vi "M2p_AD_Fifo_ToBinaryFile.vi"() -> ()   [LabVIEW 2015]
uses:
  spcm_library/spcm_gui_common.llb/element_device.ctl
  spcm_library/spcm_gui_common.llb/element_mode_fifo.ctl
  spcm_library/spcm_gui_common.llb/element_device_infos.ctl
  spcm_library/spcm_gui_m2p.llb/element_m2p_ai_channel.ctl
  spcm_library/spcm_gui_m2p.llb/element_m2p_clock.ctl
  spcm_library/spcm_gui_m2p.llb/element_m2p_ai_trigger.ctl
panel:
  out "Transferred Samples":u64=666894336
  out "Transferred Samples (MBytes)":u64=636
  in  "File Name":string="stream.dat"
  in  "Trigger Settings":T1={"Trigger Source"=0, "External Trigger"=0, "Level 0 Ext"=1500, "Ext Trig Term"=FALSE, "Channel Trigger"=0, "Level 0 Ch"=0, "Level 1 Ch"=0, "Trigger Delay (Samples)"=0} {"Channel Trigger" items=["None", "Pos. Edge", "Neg. Edge", "Any Edge", "Pos. Rearm", "Neg. Rearm", "Enter Window", "Leave Window", "In Win", "Out Win"]; "External Trigger" items=["None", "Pos. Edge", "Neg. Edge", "Any Edge", "High Level", "Low Level"]; "Trigger Source" items=["Software Trigger", "External Trigger", "Channel 0 Trigger", "Channel 1 Trigger", "Channel 2 Trigger", "Channel 3 Trigger", "Channel 4 Trigger", "Channel 5 Trigger", "Channel 6 Trigger", "Channel 7 Trigger"]; "Trigger Delay (Samples)" max=65535 step=1}
  in  "Clock Settings":T2={"Clock Mode"=0, "Sampling Rate (kHz)"=10000.0, "Clock Output"=FALSE, "Termination"=FALSE, "Ref. Clock (MHz)"=10.0, "Threshold (mV)"=1500} {"Threshold (mV)" min=-5000 max=5000; "Clock Mode" items=["Internal Clock Quartz", "External Clock", "External Reference Clock"]; "Ref. Clock (MHz)" min=0.0 max=125000.0; "Sampling Rate (kHz)" min=1.0 max=5000000.0}
  in  "AI Channel 7":T3={"Enable"=TRUE, "Input Range "=2, "Termination"=0, "Input Type"=0, "Offset"=0} {"Input Type" items=["Single-ended", "Differential"]; "Termination" items=["1 MOhm", "50 Ohm"]; "Input Range" items=["±200 mV", "±500 mV", "±1000 mV", "±2000 mV", "±5000 mV", "±10000 mV"]}
  in  "AI Channel 6":T3={"Enable"=TRUE, "Input Range "=2, "Termination"=0, "Input Type"=0, "Offset"=0} {"Input Type" items=["Single-ended", "Differential"]; "Termination" items=["1 MOhm", "50 Ohm"]; "Input Range" items=["±200 mV", "±500 mV", "±1000 mV", "±2000 mV", "±5000 mV", "±10000 mV"]}
  in  "AI Channel 5":T3={"Enable"=TRUE, "Input Range "=2, "Termination"=0, "Input Type"=0, "Offset"=0} {"Input Type" items=["Single-ended", "Differential"]; "Termination" items=["1 MOhm", "50 Ohm"]; "Input Range" items=["±200 mV", "±500 mV", "±1000 mV", "±2000 mV", "±5000 mV", "±10000 mV"]}
  in  "AI Channel 4":T3={"Enable"=TRUE, "Input Range "=2, "Termination"=0, "Input Type"=0, "Offset"=0} {"Input Type" items=["Single-ended", "Differential"]; "Termination" items=["1 MOhm", "50 Ohm"]; "Input Range" items=["±200 mV", "±500 mV", "±1000 mV", "±2000 mV", "±5000 mV", "±10000 mV"]}
  in  "AI Channel 3":T3={"Enable"=TRUE, "Input Range "=2, "Termination"=0, "Input Type"=0, "Offset"=0} {"Input Type" items=["Single-ended", "Differential"]; "Termination" items=["1 MOhm", "50 Ohm"]; "Input Range" items=["±200 mV", "±500 mV", "±1000 mV", "±2000 mV", "±5000 mV", "±10000 mV"]}
  in  "AI Channel 2":T3={"Enable"=TRUE, "Input Range "=2, "Termination"=0, "Input Type"=0, "Offset"=0} {"Input Type" items=["Single-ended", "Differential"]; "Termination" items=["1 MOhm", "50 Ohm"]; "Input Range" items=["±200 mV", "±500 mV", "±1000 mV", "±2000 mV", "±5000 mV", "±10000 mV"]}
  in  "AI Channel 1":T3={"Enable"=TRUE, "Input Range "=2, "Termination"=0, "Input Type"=0, "Offset"=0} {"Input Type" items=["Single-ended", "Differential"]; "Termination" items=["1 MOhm", "50 Ohm"]; "Input Range" items=["±200 mV", "±500 mV", "±1000 mV", "±2000 mV", "±5000 mV", "±10000 mV"]}
  in  "AI Channel 0":T3={"Enable"=TRUE, "Input Range "=2, "Termination"=0, "Input Type"=0, "Offset"=0} {"Input Type" items=["Single-ended", "Differential"]; "Termination" items=["1 MOhm", "50 Ohm"]; "Input Range" items=["±200 mV", "±500 mV", "±1000 mV", "±2000 mV", "±5000 mV", "±10000 mV"]}
  out "Device Infos":T4={"Device Name"="M2p.5942-x4", "Serial Number"=666.0, "Mem (MB)"=1024.0}
  in  "Mode Setup":T5={"Mode"=0, "Loop"=0, "Seg"=1024, "Post"=8192, "Pre"=32, "ABA"=16} {"Mode" items=["Singleshot", "Multiple Recording", "Gated Sampling", "ABA Mode"]; "ABA" min=2 max=65535 step=1; "Post" min=4 step=4; "Loop" min=8 step=4; "Pre" min=4 max=8176 step=4; "Seg" min=8 step=4}
  in  "Device":T6 {"Device" items=["Card", "digitizerNETBOX"]}
  out "Fillsize Fifo":i32(slide)=62 scale=0.0..1000.0
  out "Status":string="Stopped"
  in  "Quit Button":bool
  in  "Force Trigger Button":bool
  in  "Start Button":bool
  in  "Stop Button":bool
  # "M2p AD FIFO Example"
  # "Mode Settings"
  # "Trigger Settings"
  # "Range"
  # "Term"
  # "Type"
  # "Offset"
  # "Ch0"
  # "Ch1"
  # "Ch2"
  # "Clock Settings"
  # "Ch3"
  # "Ch4"
  # "Ch5"
  # "Ch6"
  # "Ch7"
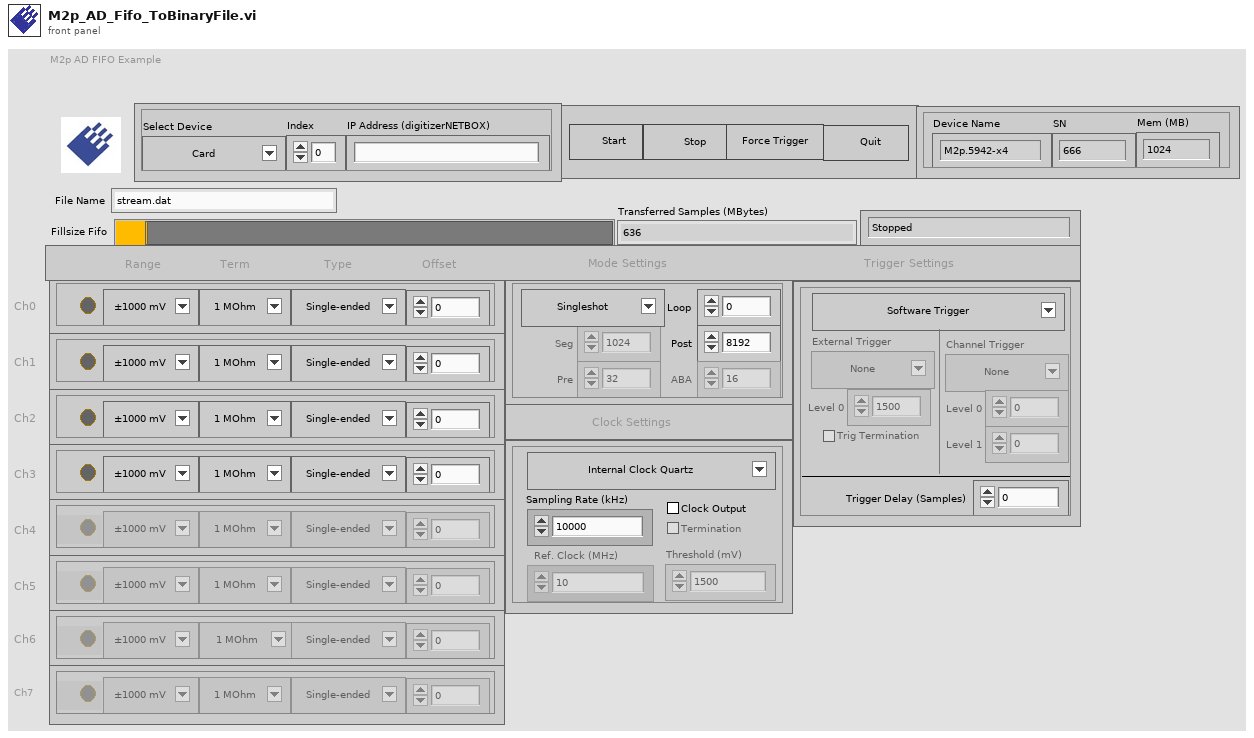
[diagram p1: front panel]
types:
  T1 = typedef "element_m2p_ai_trigger.ctl" = cluster{"Trigger Source":u16, "External Trigger":u16, "Level 0 Ext":i32, "Ext Trig Term":bool, "Channel Trigger":u16, "Level 0 Ch":i32, "Level 1 Ch":i32, "Trigger Delay (Samples)":u32}
  T2 = typedef "element_m2p_clock.ctl" = cluster{"Clock Mode":u16, "Sampling Rate (kHz)":dbl, "Clock Output":bool, "Termination":bool, "Ref. Clock (MHz)":dbl, "Threshold (mV)":i32}
  T3 = typedef "element_m2p_ai_channel.ctl" = cluster{"Enable":bool, "Input Range ":u16, "Termination":u16, "Input Type":u16, "Offset":i32}
  T4 = typedef "element_device_infos.ctl" = cluster{"Device Name":string, "Serial Number":dbl, "Mem (MB)":dbl}
  T5 = typedef "element_mode_fifo.ctl" = cluster{"Mode":u16, "Loop":u32, "Seg":u32, "Post":u32, "Pre":u32, "ABA":u32}
  T6 = typedef "element_device.ctl" = cluster{"Index":dbl, "IP Address":string, "Device":u16}
  T7 = enum16{"Idle", "Init", "Stop", "Write Setup", "Start", "Acquire", "Read Data", "Quit"}
  T8 = cluster{"Card Type":i32, "Inst Mem (high part)":i32, "Inst Mem (low part)":i32, "Serial Number":i32, "Function Type":i32, "Installed Features":i32, "Base Card Version":i32, "Module Version":i32, "Extension Version":i32, "Production Date":i32, "Max Sampling Rate":i32, "Max Channels":i32, "Demo Card":i32}
  T9 = cluster{"Card Name":string, "SN":i32, "Mem (MB)":i32}
  T10 = cluster{"AI Channels":i32, "AI Ranges":i32, "Input Ranges (mV)":i32[], "Programmable Offset":i32, "Termination Available":bool, "SE/Diff switchable":bool, "Offset in per cent/mV":bool, "Offset Calibration":bool, "Gain Calibration":bool, "Offset with open inputs":bool, "AI Range Strings[]":string[], "Bit Resolution":i32, "AC Coupling available":bool, "BW Limit available":bool, "AI Path count":i32}
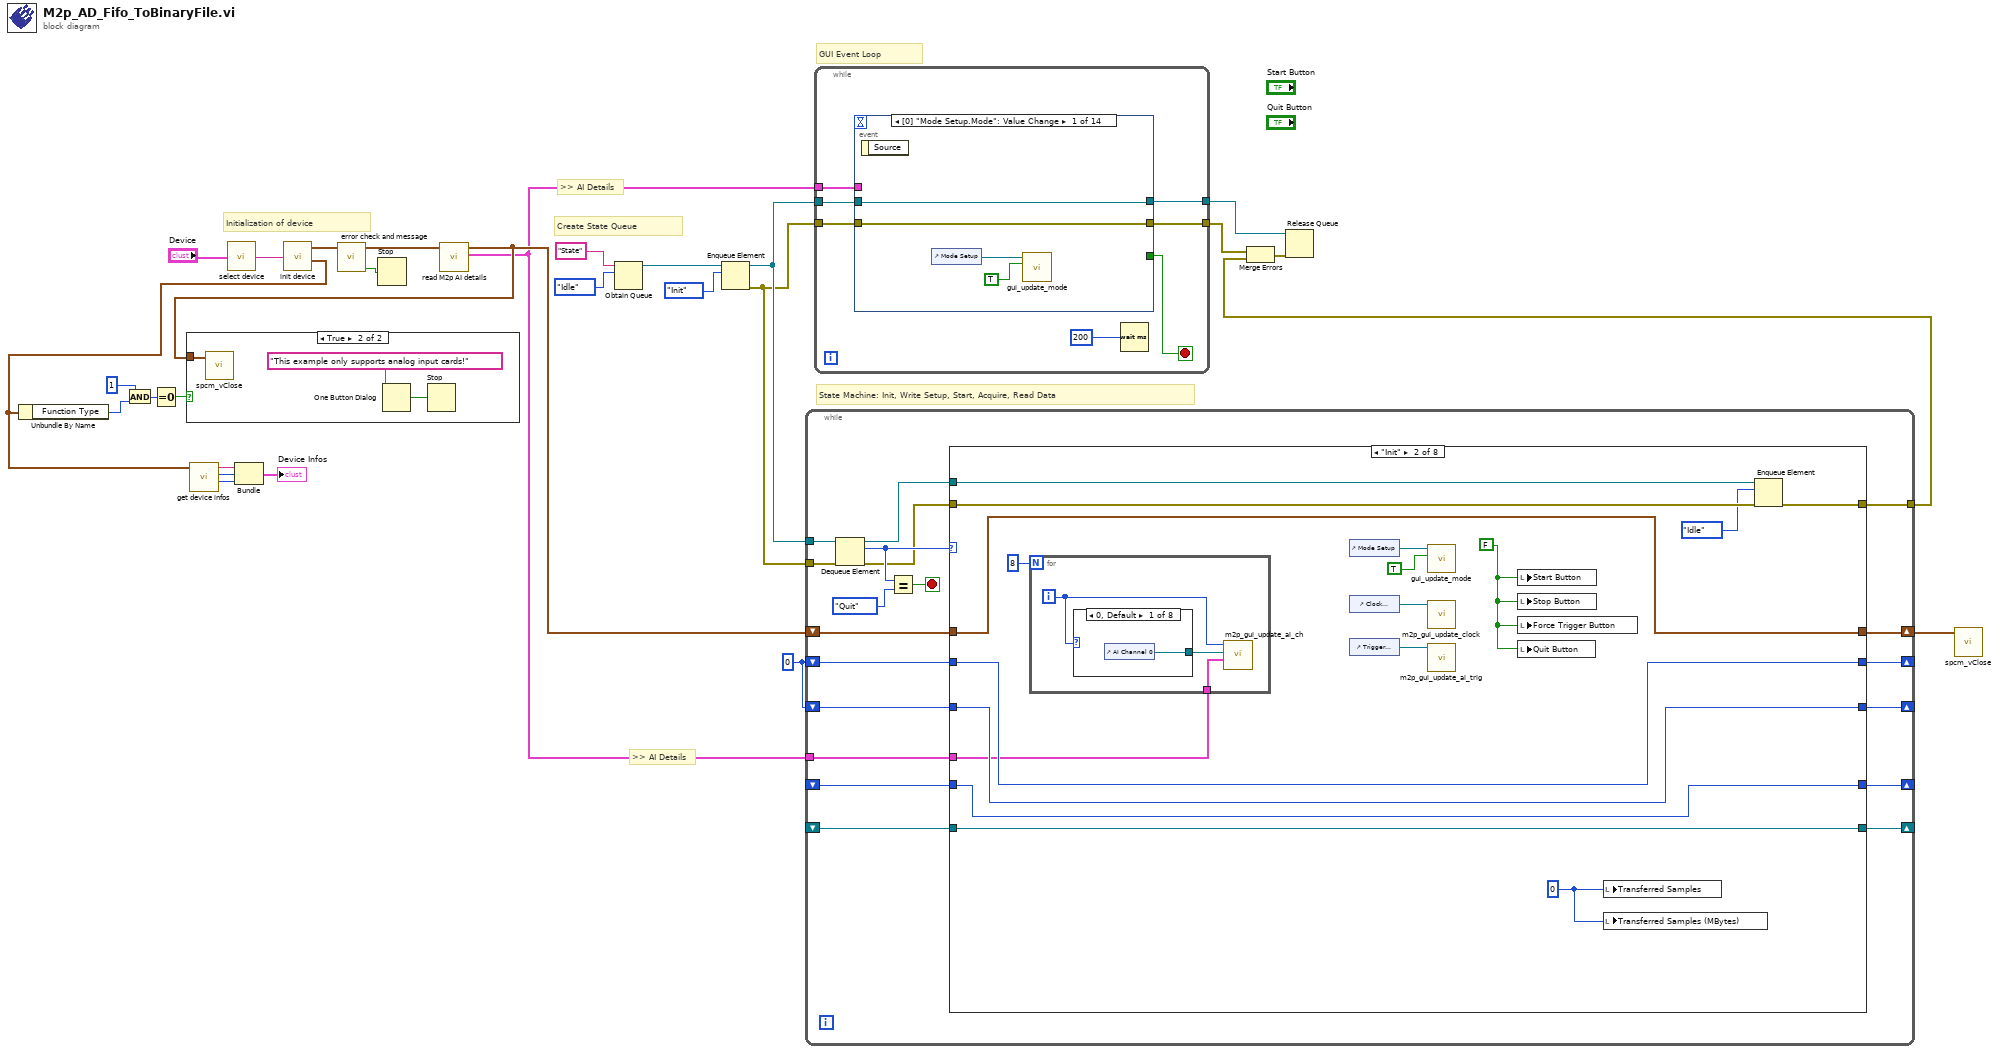
[diagram p0: block diagram]
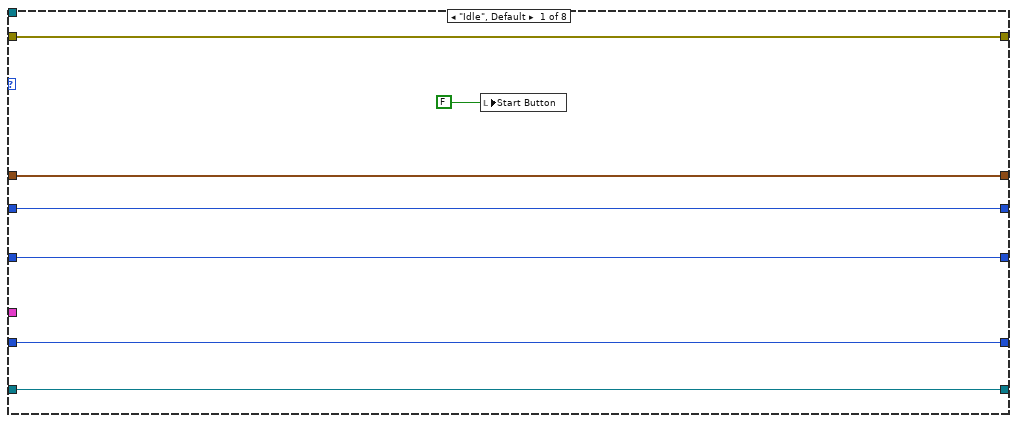
[diagram p3: hidden frame]
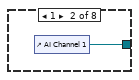
[diagram p4: hidden frame]
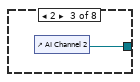
[diagram p5: hidden frame]
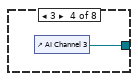
[diagram p6: hidden frame]
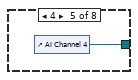
[diagram p7: hidden frame]
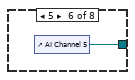
[diagram p8: hidden frame]
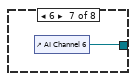
[diagram p9: hidden frame]
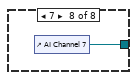
[diagram p10: hidden frame]
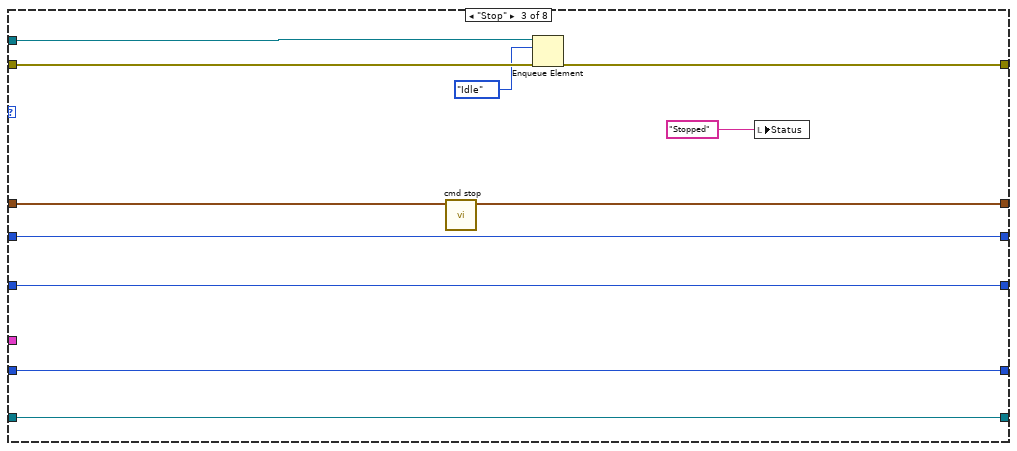
[diagram p11: hidden frame]
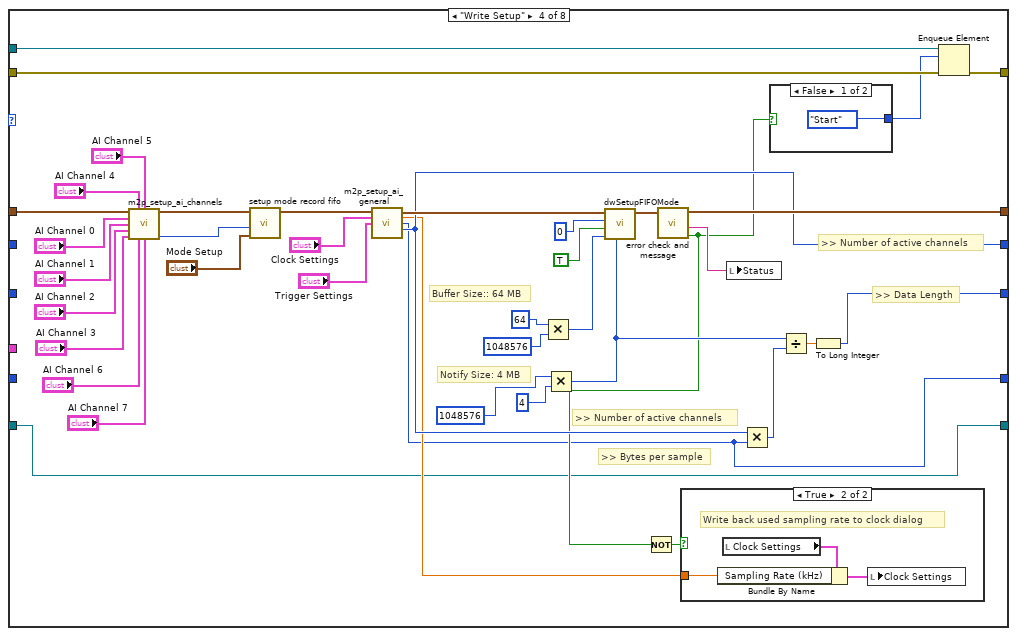
[diagram p12: hidden frame]
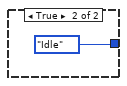
[diagram p14: hidden frame]
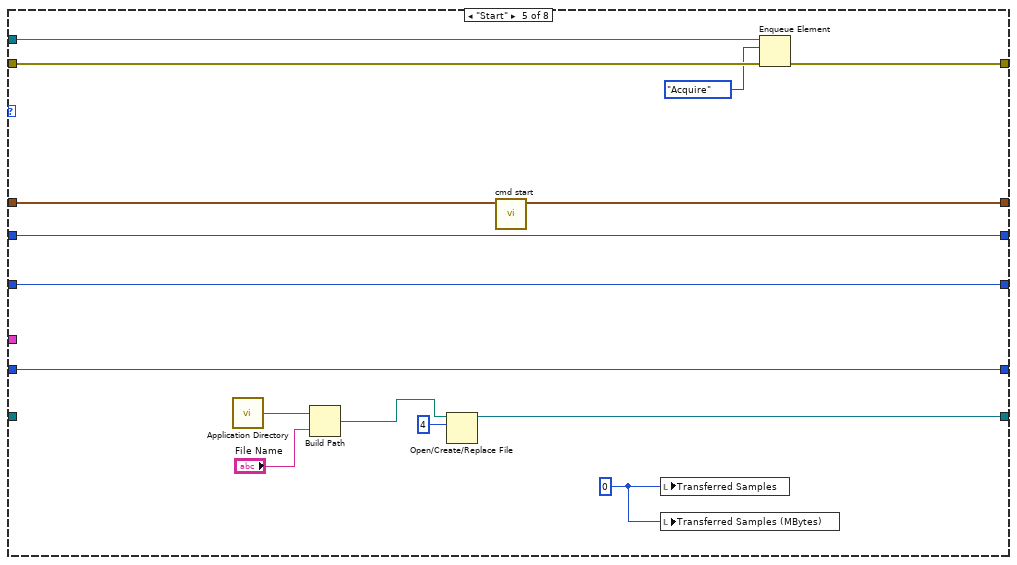
[diagram p15: hidden frame]
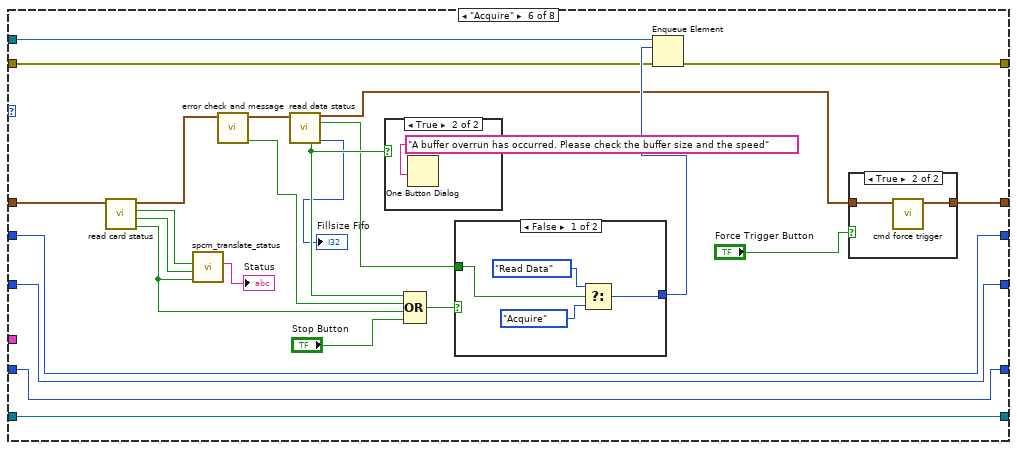
[diagram p16: hidden frame]
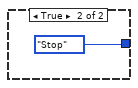
[diagram p18: hidden frame]
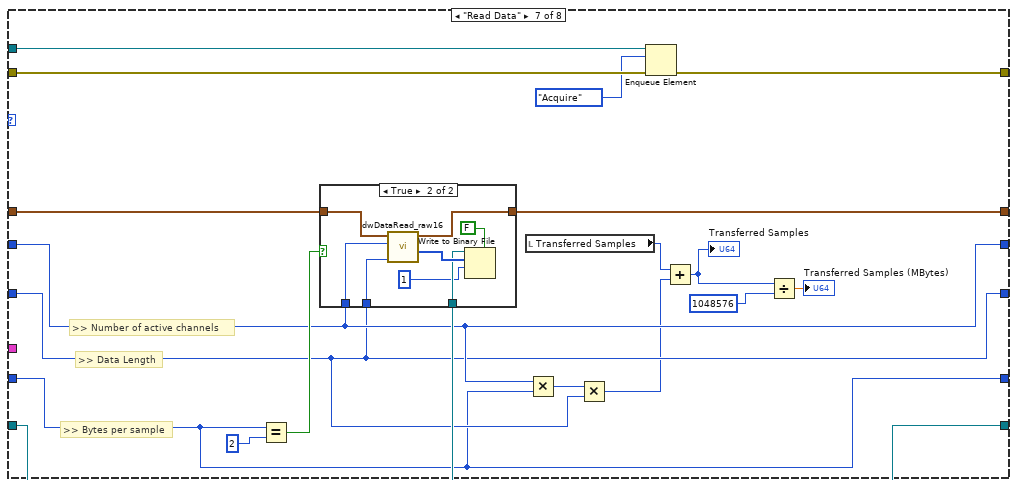
[diagram p20: hidden frame]
diagram:
  w6 = 0
  # ">> AI Details"
  # ">> AI Details"
  # "Initialization of device"
  # "Create State Queue"
  # "State Machine: Init, Write Setup, Start, Acquire, Read Data"
  # "GUI Event Loop"
  n1 = call "select device.vi"("Device"="Device") -> ("device string"=w28:string)  [unwired: 4 in]
  n2 = call "init device.vi"("Device String"=w28) -> ("Card Info Out"=w27:cluster{"Card Handle":u64, "Error Code":u32}, "Card Information"=w14:T8)  [unwired: 4 in]
  n3 = Unbundle By Name(w14) -> ("Function Type"=w18:i32)
  n4 = And(x=1, y=w18) -> (x .and. y?=w17:i32)
  n5 = Equal To 0?(x=w17) -> (x = 0?=w15:bool)
  n6 = call "get device infos.vi"("Card Information"=w14) -> ("Mem (MB)"=w21:i32, "SN"=w20:i32, "Card Name"=w19:string)  [unwired: 8 in]
  n7 = Bundle("Card Name"=w19, "SN"=w20, "Mem (MB)"=w21) -> (→"Device Infos":T9)  [unwired: 1 in]
  n8 = call "error check and message.vi"("Card Info In"=w27) -> ("Error occurred"=w26:bool, "Card Info Out"=w4:cluster{"Card Handle":u64, "Error Code":u32})  [unwired: 4 in, 1 out]
  n9 = Stop(stop? (T)=w26) -> ()
  n10 = call "read M2p AI details.vi"("Card Info In"=w4) -> ("AI Details"=w2:T10, "Card Info Out"=w3:cluster{"Card Handle":u64, "Error Code":u32})  [unwired: 5 in]
  n11 = case shown="True" w15 {
    tunnel: w3 -> [_ w29]
    frame False {
    }
    frame True {
      n12 = call "spcm_vClose.vi"("Card Info In"=w29) -> ()  [unwired: 7 in]
      n13 = One Button Dialog(message="This example only supports analog input cards!") -> (true=w30:bool)  [unwired: 1 in]
      n14 = Stop(stop? (T)=w30) -> ()
    }
  }
  n15 = Obtain Queue(name (unnamed)="State", element data type=T7."Idle") -> (queue out=w23:refnum<queue>)  [unwired: 3 in, 2 out]
  n16 = Enqueue Element(queue=w23, element=T7."Init") -> (queue out=w24:refnum<queue>, error out=w9:errorcluster)  [unwired: 2 in, 1 out]
  n17 = while {
    tunnel: w24 -> [w50]
    shift-right: [w48] -> w22
    shift-left: w3 -> [w49]
    shift-right: [w43] -> _
    shift-left: w6 -> [w44]
    tunnel: [w42] -> w12
    tunnel: w9 -> [w41]
    shift-right: [w38] -> _
    shift-left: w6 -> [w37]
    tunnel: w2 -> [w36]
    shift-right: [w35] -> _
    shift-left: _ -> [w34]
    shift-right: [w33] -> _
    shift-left: _ -> [w32]
    stop <- w46 stop-if-true
    n18 = Dequeue Element(queue=w50, error in (no error)=w41) -> (queue out=w45:refnum<queue>, element=w47:T7, error out=w40:errorcluster)  [unwired: 1 in, 1 out]
    n19 = Equal?(x=w47, y=T7."Quit") -> (x = y?=w46:bool)
    n20 = case shown="\"Init\"" w47 {
      tunnel: w49 -> [w57 w67 w93 w112 w155 w170 w203 w225]
      tunnel: [w57 w67 w92 w133 w154 w177 w202 w224] -> w48
      tunnel: w45 -> [_ w74 w96 w136 w152 w175 w207 _]
      tunnel: w44 -> [w56 w68 w91 _ w156 w174 w198 w231]
      tunnel: [w56 w68 w91 w115 w156 w174 w198 w231] -> w43
      tunnel: [w55 w72 w94 w134 w151 w172 w206 w232] -> w42
      tunnel: w40 -> [w55 w71 w95 w135 w153 w171 w205 w232]
      tunnel: [w53 w69 w90 w123 w149 w158 w196 w230] -> w38
      tunnel: w37 -> [w53 w69 w90 _ w149 w158 w196 w230]
      tunnel: w36 -> [_ w64 _ _ _ _ _ _]
      tunnel: [w52 w60 w87 w98 w143 w159 w199 w229] -> w35
      tunnel: w34 -> [w52 w60 w87 w98 _ w159 w199 w229]
      tunnel: [w51 w59 w86 w97 w142 w157 w190 w228] -> w33
      tunnel: w32 -> [w51 w59 w86 _ w142 w157 w190 w228]
      frame "Idle", Default {
        n21 = local write "Start Button"(FALSE) -> ()
      }
      frame "Init" {
        w61 = 0
        w73 = FALSE
        n22 = for {
          N: 8 -> [_]
          tunnel: w64 -> [w75]
          i -> [w77]
          n23 = case shown="0, Default" w77 {
            tunnel: [w78 w79 w80 w81 w82 w83 w84 w85] -> w76
            frame 0, Default {
              n24 = control-ref of="AI Channel 0"() -> (w78:refnum<vi>)
            }
            frame 1 {
              n25 = control-ref of="AI Channel 1"() -> (w79:refnum<vi>)
            }
            frame 2 {
              n26 = control-ref of="AI Channel 2"() -> (w80:refnum<vi>)
            }
            frame 3 {
              n27 = control-ref of="AI Channel 3"() -> (w81:refnum<vi>)
            }
            frame 4 {
              n28 = control-ref of="AI Channel 4"() -> (w82:refnum<vi>)
            }
            frame 5 {
              n29 = control-ref of="AI Channel 5"() -> (w83:refnum<vi>)
            }
            frame 6 {
              n30 = control-ref of="AI Channel 6"() -> (w84:refnum<vi>)
            }
            frame 7 {
              n31 = control-ref of="AI Channel 7"() -> (w85:refnum<vi>)
            }
          }
          n32 = call "m2p_gui_update_ai_ch.vi"("AI Details"=w75, "Cluster Referenz"=w76, "Channel Index"=w77) -> ()  [unwired: 9 in]
        }
        n33 = control-ref of="Mode Setup"() -> (w66:refnum<vi>)
        n34 = control-ref of="Clock Settings"() -> (w63:refnum<vi>)
        n35 = control-ref of="Trigger Settings"() -> (w62:refnum<vi>)
        n36 = call "gui_update_mode.vi"("Fifo Mode"=TRUE, "Referenz Mode Settings"=w66) -> ()  [unwired: 10 in]
        n37 = call "m2p_gui_update_clock.vi"("Cluster Reference"=w63) -> ()  [unwired: 11 in]
        n38 = call "m2p_gui_update_ai_trig.vi"("Trigger Settings Reference"=w62) -> ()  [unwired: 10 in]
        n39 = local write "Start Button"(w73) -> ()
        n40 = local write "Stop Button"(w73) -> ()
        n41 = local write "Force Trigger Button"(w73) -> ()
        n42 = local write "Quit Button"(w73) -> ()
        n43 = local write "Transferred Samples"(w61) -> ()
        n44 = local write "Transferred Samples (MBytes)"(w61) -> ()
        n45 = Enqueue Element(queue=w74, element=T7."Idle", error in (no error)=w71) -> (error out=w72:errorcluster)  [unwired: 1 in, 2 out]
      }
      frame "Stop" {
        n46 = call "cmd stop.vi"("Card Info In"=w93) -> ("Card Info Out"=w92:cluster{"Card Handle":u64, "Error Code":u32})  [unwired: 6 in]
        n47 = Enqueue Element(queue=w96, element=T7."Idle", error in (no error)=w95) -> (error out=w94:errorcluster)  [unwired: 1 in, 2 out]
        n48 = local write "Status"("Stopped") -> ()
      }
      frame "Write Setup" {
        # ">> Data Length"
        # ">> Number of active channels"
        # ">> Bytes per sample"
        # ">> Number of active channels"
        # "Buffer Size:: 64 MB"
        # "Notify Size: 4 MB"
        n49 = call "m2p_setup_ai_channels.vi"("Card Info In"=w112, "AI Channel 4"="AI Channel 4", "AI Channel 5"="AI Channel 5", "AI Channel 0"="AI Channel 0", "AI Channel 1"="AI Channel 1", "AI Channel 2"="AI Channel 2", "AI Channel 3"="AI Channel 3", "AI Channel 6"="AI Channel 6", "AI Channel 7"="AI Channel 7") -> ("Card Info Out"=w113:cluster{"Card Handle":u64, "Error Code":u32}, "ChMask"=w103:i32)  [unwired: 5 in]
        n50 = call "setup mode record fifo.vi"("Mode Fifo Setup"="Mode Setup", "Channel Mask Low"=w103, "Card Info In"=w113) -> ("Card Info Out"=w117:cluster{"Card Handle":u64, "Error Code":u32})  [unwired: 2 in, 2 out]
        n51 = call "m2p_setup_ai_general.vi"("Card Info In"=w117, "Clock Settings"="Clock Settings", "Trigger Settings"="Trigger Settings") -> ("Card Info Out"=w116:cluster{"Card Handle":u64, "Error Code":u32}, "Used Sampling Rate (kS)"=w114:dbl, "Bytes Per Sample"=w97:i32, "Channel Count"=w115:i32)  [unwired: 9 in]
        n52 = Multiply(x=u32 64 ("Channel MaskOut"), y=u32 1048576 ("Channel MaskOut")) -> (x*y=w126:u32)
        n53 = Multiply(x=u32 1048576 ("Channel MaskOut"), y=u32 4 ("Channel MaskOut")) -> (x*y=w120:u32)
        n54 = call "dwSetupFIFOMode.vi"("Notify (Bytes)"=w120, "Bufferlength (Bytes)"=w126, "Allocate"=TRUE, "Buffertype (0=data, 1=TS, 2=ABA)"=0, "Card Info In"=w116) -> ("Card Info Out"=w130:cluster{"Card Handle":u64, "Error Code":u32})  [unwired: 4 in]
        n55 = call "error check and message.vi"("Card Info In"=w130) -> ("Error occurred"=w99:bool, "Error Message"=w131:string, "Card Info Out"=w133:cluster{"Card Handle":u64, "Error Code":u32})  [unwired: 4 in]
        n56 = Not(x=w99) -> (.not. x?=w100:bool)
        n57 = case shown="True" w100 {
          tunnel: w114 -> [_ w139]
          frame False {
          }
          frame True {
            # "Write back used sampling rate to clock dialog"
            n58 = local read "Clock Settings"() -> (w138:T2)
            n59 = Bundle By Name(cluster=w138, "Sampling Rate (kHz)"=w139) -> (w137:T2)
            n60 = local write "Clock Settings"(w137) -> ()
          }
        }
        n61 = local write "Status"(w131) -> ()
        n62 = Multiply(x=w115, y=w97) -> (x*y=w125:i32)
        n63 = case shown="False" w99 {
          tunnel: [T7."Start" T7."Idle"] -> w132
          frame False {
          }
          frame True {
          }
        }
        n64 = Divide(x=w120, y=w125) -> (x/y=w124:dbl)
        n65 = To Long Integer(number=w124) -> (32bit integer=w123:i32)
        n66 = Enqueue Element(queue=w136, element=w132, error in (no error)=w135) -> (error out=w134:errorcluster)  [unwired: 1 in, 2 out]
      }
      frame "Start" {
        w144 = 0
        n67 = call <vilib>:"Application Directory.vi"() -> ("Application Directory"=w146:path)
        n68 = Build Path(base path=w146, name or relative path="File Name") -> (appended path=w148:path)
        n69 = Open/Create/Replace File(file path (use dialog)=w148, operation (0:open)=4) -> (refnum out=w143:refnum<file>)  [unwired: 4 in, 2 out]
        n70 = call "cmd start.vi"("Card Info In"=w155) -> ("Card Info Out"=w154:cluster{"Card Handle":u64, "Error Code":u32})  [unwired: 6 in]
        n71 = local write "Transferred Samples"(w144) -> ()
        n72 = local write "Transferred Samples (MBytes)"(w144) -> ()
        n73 = Enqueue Element(queue=w152, element=T7."Acquire", error in (no error)=w153) -> (error out=w151:errorcluster)  [unwired: 1 in, 2 out]
      }
      frame "Acquire" {
        n74 = call "read card status.vi"("Card Info In"=w170) -> ("Card ready"=w162:bool, "Trigger detected"=w179:bool, "Pretrigger full"=w180:bool, "Card Info Out"=w169:cluster{"Card Handle":u64, "Error Code":u32})  [unwired: 3 in]
        n75 = call "spcm_translate_status.vi"("Ready"=w162, "Trigger"=w179, "Pretrigger"=w180) -> ("Text"=→"Status":string)  [unwired: 4 in]
        n76 = call "error check and message.vi"("Card Info In"=w169) -> ("Error occurred"=w164:bool, "Card Info Out"=w168:cluster{"Card Handle":u64, "Error Code":u32})  [unwired: 4 in, 1 out]
        n77 = call "read data status.vi"("Card Info In"=w168) -> ("Card Info Out"=w167:cluster{"Card Handle":u64, "Error Code":u32}, "Next block ready"=w161:bool, "Overrun"=w165:bool, "Fillsize o/oo"=→"Fillsize Fifo":i32)  [unwired: 10 in, 1 out]
        n78 = case shown="True" w165 {
          frame False {
          }
          frame True {
            n79 = One Button Dialog(message="A buffer overrun has occurred. Please check the buffer size and the speed") -> ()  [unwired: 1 in, 1 out]
          }
        }
        n80 = Compound Arithmetic op=OR(w165, w164, w162, "Stop Button") -> (w166:bool)
        n81 = case shown="False" w166 {
          tunnel: [w182 T7."Stop"] -> w178
          tunnel: w161 -> [w185 _]
          frame False {
            n82 = Select(t=T7."Read Data", s=w185, f=T7."Acquire") -> (s? t:f=w182:T7)
          }
          frame True {
          }
        }
        n83 = Enqueue Element(queue=w175, element=w178, error in (no error)=w171) -> (error out=w172:errorcluster)  [unwired: 1 in, 2 out]
        n84 = case shown="True" "Force Trigger Button" {
          tunnel: w167 -> [w187 w189]
          tunnel: [w187 w188] -> w177
          frame False {
          }
          frame True {
            n85 = call "cmd force trigger.vi"("Card Info In"=w189) -> ("Card Info Out"=w188:cluster{"Card Handle":u64, "Error Code":u32})  [unwired: 6 in]
          }
        }
      }
      frame "Read Data" {
        # ">> Bytes per sample"
        # ">> Data Length"
        # ">> Number of active channels"
        n86 = Equal?(x=w190, y=2) -> (x = y?=w200:bool)
        n87 = case shown="True" w200 {
          tunnel: w203 -> [w214 w223]
          tunnel: w198 -> [w213 w222]
          tunnel: w196 -> [w212 w221]
          tunnel: [w215 w220] -> w202
          tunnel: w199 -> [w210 w218]
          frame False {
            n88 = call "dwDataRead_raw8.vi"("Length (Samples per Channel)"=w212, "Channel Count"=w213, "Card Info In"=w214) -> ("RAW Data"=w209:i8[], "Card Info Out"=w215:cluster{"Card Handle":u64, "Error Code":u32})  [unwired: 7 in]
            n89 = Write to Binary File(file (use dialog)=w210, data=w209, 5:FALSE, 9:1) -> ()  [unwired: 2 in, 3 out]
          }
          frame True {
            n90 = call "dwDataRead_raw16.vi"("Length (Samples per Channel)"=w221, "Channel Count"=w222, "Card Info In"=w223) -> ("RAW Data"=w219:i16[], "Card Info Out"=w220:cluster{"Card Handle":u64, "Error Code":u32})  [unwired: 7 in]
            n91 = Write to Binary File(file (use dialog)=w218, data=w219, 5:FALSE, 9:1) -> ()  [unwired: 2 in, 3 out]
          }
        }
        n92 = local read "Transferred Samples"() -> (w195:u64)
        n93 = Multiply(x=w198, y=w190) -> (x*y=w197:i32)
        n94 = Multiply(x=w197, y=w196) -> (x*y=w194:i32)
        n95 = Enqueue Element(queue=w207, element=T7."Acquire", error in (no error)=w205) -> (error out=w206:errorcluster)  [unwired: 1 in, 2 out]
        n96 = Add(x=w195, y=w194) -> (x+y=w191:u64)
        "Transferred Samples" <- w191
        n97 = Divide(x=w191, y=u32 1048576 ("Channel MaskOut")) -> (x/y=→"Transferred Samples (MBytes)":dbl)
      }
      frame "Quit" {
        n98 = call "dwSetupFIFOMode.vi"("Allocate"=FALSE, "Buffertype (0=data, 1=TS, 2=ABA)"=0, "Card Info In"=w225) -> ("Card Info Out"=w224:cluster{"Card Handle":u64, "Error Code":u32})  [unwired: 6 in]
      }
    }
  }
  n99 = while {
    tunnel: w24 -> [w237]
    tunnel: [w238] -> w10
    tunnel: [w234] -> w13
    tunnel: w9 -> [w235]
    tunnel: w2 -> [w233]
    stop <- w236 stop-if-true
    n100 = event shown="[0] \"Mode Setup.Mode\": Value Change" {
      selector: _ -> [_ _ _ _ _ _ _ _ _ _ _ _ _ _]
      dyn-events: _ -> [_ _ _ _ _ _ _ _ _ _ _ _ _ _]
      timeout: _ -> [_ _ _ _ _ _ _ _ _ _ _ _ _ _]
      tunnel: [_ _ _ _ _ _ _ _ _ _ _ _ _ TRUE] -> w236
      tunnel: [w243 w246 w249 w254 w259 w264 w269 _ _ _ _ w286 w292 w297] -> w238
      tunnel: w237 -> [w243 w246 w249 w254 w259 w264 w269 _ _ _ _ w285 w291 w298]
      tunnel: [w242 w245 w248 w253 w258 w263 w268 _ _ _ _ w283 w288 w295] -> w234
      tunnel: w235 -> [w242 w245 w248 w253 w258 w263 w268 _ _ _ _ w284 w289 w294]
      tunnel: w233 -> [_ _ _ w250 w255 w260 w265 w270 w273 w276 w279 _ _ _]
      event Value Change {
        n101 = event-data ("Ereignisdatenknoten")() -> ()  [unwired: 1 in, 1 out]
        n102 = control-ref of="Mode Setup"() -> (w241:refnum<vi>)
        n103 = call "gui_update_mode.vi"("Fifo Mode"=TRUE, "Referenz Mode Settings"=w241) -> ()  [unwired: 10 in]
      }
      event Value Change {
        n104 = event-data() -> ()  [unwired: 1 in, 1 out]
        n105 = control-ref of="Clock Settings"() -> (w244:refnum<vi>)
        n106 = call "m2p_gui_update_clock.vi"("Cluster Reference"=w244) -> ()  [unwired: 11 in]
      }
      event Value Change {
        n107 = event-data() -> ()  [unwired: 1 in, 1 out]
        n108 = control-ref of="Trigger Settings"() -> (w247:refnum<vi>)
        n109 = call "m2p_gui_update_ai_trig.vi"("Trigger Settings Reference"=w247) -> ()  [unwired: 10 in]
      }
      event Value Change {
        n110 = event-data() -> ()  [unwired: 1 in, 1 out]
        n111 = control-ref of="AI Channel 0"() -> (w251:refnum<vi>)
        n112 = call "m2p_gui_update_ai_ch.vi"("AI Details"=w250, "Cluster Referenz"=w251, "Channel Index"=0) -> ()  [unwired: 9 in]
      }
      event Value Change {
        n113 = event-data() -> ()  [unwired: 1 in, 1 out]
        n114 = control-ref of="AI Channel 1"() -> (w256:refnum<vi>)
        n115 = call "m2p_gui_update_ai_ch.vi"("AI Details"=w255, "Cluster Referenz"=w256, "Channel Index"=1) -> ()  [unwired: 9 in]
      }
      event Value Change {
        n116 = event-data() -> ()  [unwired: 1 in, 1 out]
        n117 = control-ref of="AI Channel 2"() -> (w261:refnum<vi>)
        n118 = call "m2p_gui_update_ai_ch.vi"("AI Details"=w260, "Cluster Referenz"=w261, "Channel Index"=2) -> ()  [unwired: 9 in]
      }
      event Value Change {
        n119 = event-data() -> ()  [unwired: 1 in, 1 out]
        n120 = control-ref of="AI Channel 3"() -> (w266:refnum<vi>)
        n121 = call "m2p_gui_update_ai_ch.vi"("AI Details"=w265, "Cluster Referenz"=w266, "Channel Index"=3) -> ()  [unwired: 9 in]
      }
      event Value Change {
        n122 = event-data() -> ()  [unwired: 1 in, 1 out]
        n123 = control-ref of="AI Channel 4"() -> (w271:refnum<vi>)
        n124 = call "m2p_gui_update_ai_ch.vi"("AI Details"=w270, "Cluster Referenz"=w271, "Channel Index"=4) -> ()  [unwired: 9 in]
      }
      event Value Change {
        n125 = event-data() -> ()  [unwired: 1 in, 1 out]
        n126 = control-ref of="AI Channel 5"() -> (w274:refnum<vi>)
        n127 = call "m2p_gui_update_ai_ch.vi"("AI Details"=w273, "Cluster Referenz"=w274, "Channel Index"=5) -> ()  [unwired: 9 in]
      }
      event Value Change {
        n128 = event-data() -> ()  [unwired: 1 in, 1 out]
        n129 = control-ref of="AI Channel 6"() -> (w277:refnum<vi>)
        n130 = call "m2p_gui_update_ai_ch.vi"("AI Details"=w276, "Cluster Referenz"=w277, "Channel Index"=6) -> ()  [unwired: 9 in]
      }
      event Value Change {
        n131 = event-data() -> ()  [unwired: 1 in, 1 out]
        n132 = control-ref of="AI Channel 7"() -> (w280:refnum<vi>)
        n133 = call "m2p_gui_update_ai_ch.vi"("AI Details"=w279, "Cluster Referenz"=w280, "Channel Index"=7) -> ()  [unwired: 9 in]
      }
      event "Start Button": Value Change {
        n134 = event-data() -> ()  [unwired: 1 in, 1 out]
        n135 = Enqueue Element(queue=w285, element=T7."Write Setup", error in (no error)=w284) -> (queue out=w286:refnum<queue>, error out=w283:errorcluster)  [unwired: 1 in, 1 out]
      }
      event "Stop Button": Value Change {
        n136 = event-data() -> ()  [unwired: 1 in, 1 out]
        n137 = local write "Start Button"(FALSE) -> ()
        n138 = Enqueue Element(queue=w291, element=T7."Stop", error in (no error)=w289) -> (queue out=w292:refnum<queue>, error out=w288:errorcluster)  [unwired: 1 in, 1 out]
      }
      event "Quit Button": Value Change {
        n139 = event-data() -> ()  [unwired: 1 in, 1 out]
        n140 = Enqueue Element(queue=w298, element=T7."Quit", error in (no error)=w294) -> (queue out=w297:refnum<queue>, error out=w295:errorcluster)  [unwired: 1 in, 1 out]
      }
    }
    n141 = Wait (ms)(milliseconds to wait=200) -> ()  [unwired: 1 out]
  }
  n142 = Merge Errors(w13, w12) -> (w11:errorcluster)
  n143 = Release Queue(queue=w10, error in (no error)=w11) -> ()  [unwired: 1 in, 3 out]
  n144 = call "spcm_vClose.vi"("Card Info In"=w22) -> ()  [unwired: 7 in]
